vi "OpenByRefnumAndRunFP.vi"(0 "VI refnum":refnum<vi>, 5 "Wait until VI done?":bool caption="Wait until VI done? (F)", 7 "Auto dispose VI refnum?":bool=TRUE caption="Auto dispose VI refnum? (T)", 9 "Reentrancy mode":T2=enum."Auto" caption="Reentrancy mode (Auto)", 11 "Error in":errorcluster caption="Error in (no error)", 12 "Control names":string[](array[string]) caption="Control names (none)", 13 "Control values":variant[](array[variant]) caption="Control values (none)") -> (3 "VI refnum opened?":bool, 4 "VI refnum out":refnum<vi>, 6 "VI running?":bool, 8 "Last execution state":T1(ring), 10 "VI refnum opened as reentrant?":bool, 14 "Control values set?":bool, 15 "Error out":errorcluster)   [LabVIEW 2017, in "VILauncher.lvlib"]
doc: "Opens a reference to a dynamic VI either specified by path (<B>VI path</B>) or by reference (<B>VI refnum</B>), runs the dynamic VI, and returns the reference to it in <B>VI refnum out</B>.\n\nThis function will wait until the dynamic VI is done if <B>Wait until VI done?</B> is True (default is False), and it will auto dispose the dynamic VI reference (hand it over to the running dynamic VI) if <B>Auto dispose VI refnum?</B> is True. Note that if this function fails to run the dynamic VI, it will close the opened VI reference itself, in which case <B>VI refnum opened?</B> will be False and <B>VI refnum out</B> will be invalid.\n\nUse the optional <B>Reentrancy mode</B> input to specify whether the dynamic VI should be opened as a reentrant or a non-reentrant instance. Set this to Auto (default) to first try as reentrant, and if that fails, as non-reentrant. The <B>VI refnum opened as reentrant?</B> output will reflect the eventual instantiation mode.\n\nThe <B>VI running?</B> output will only be True if the dynamic VI's <B>Last execution state</B> is \"Run top level\". <B>VI running?</B> can be False even if the dynamic VI ran successfully - it might just have finished before this VI finished.\n\nOptionally you can send input data to the dynamic VI when running it using one of two modes; Right click this VI and use the Select Type menu to choose input data transfer mode:\n\nInput data via front panel\n-------------------------------\nSet data on the front panel of the dynamic VI before running it by wiring <B>Control names</B> and <B>Control values</B>. <B>Control values set?</B> will be True only if all <B>Control names</B> were valid.\n\nInput data via block diagram\n----------------------------------\nTransmit data to the dynamic VI after it has started by wiring <B>Input data names</B> and <B>Input data values</B>. If you use this mode the dynamic VI must use the WaitForInputData function to read the input data on the block diagram. The read in the dynamic VI must be finished before <B>Input data timeout</B> runs out. Set this timeout value to -1 (default) to wait indefinitely. If timeout does occur, <B>Input data timed out?</B> will be True. <B>Input data delivered?</B> will be True only if input data was in fact transmitted to the dynamic VI without any errors.\n\n<B>NOTE 1:</B> When using the 'Input data via block diagram' mode the dynamic VI must use the WaitForInputData function even if you send zero input data. To avoid this requirement for the dynamic VI when not passing any input data, please use the 'Input data via front panel' mode in this case.\n\n<B>NOTE 2:</B> The dynamic VI must have its front panel available at runtime for this function to work. The simplest way to ensure this, which also works in a built application without additional steps to be taken, is by enabling \"Show front panel when called\" in the \"Window Appearance\" section of the dynamic VI Properties.\n\nThis VI is reentrant, and it will only run if there is no error on <B>Error in</B>.\n\nSteen Schmidt\nGPower\n2/1 2013"
uses:
  VILauncher.lvlib
  Typedefs/ReentrancyMode.ctl
panel:
  # "Copyright © 2013\nGPower\nSee enclosed license file for terms and conditions"
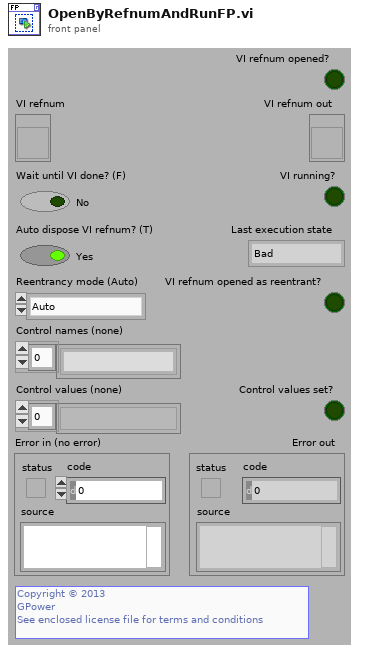
[diagram p1: front panel]
types:
  T1 = enum32{"Bad", "Idle", "Run top level", "Running"}
  T2 = typedef "VILauncher.lvlib/ReentrancyMode.ctl" = enum16{"Reentrant", "Non-reentrant", "Auto"}
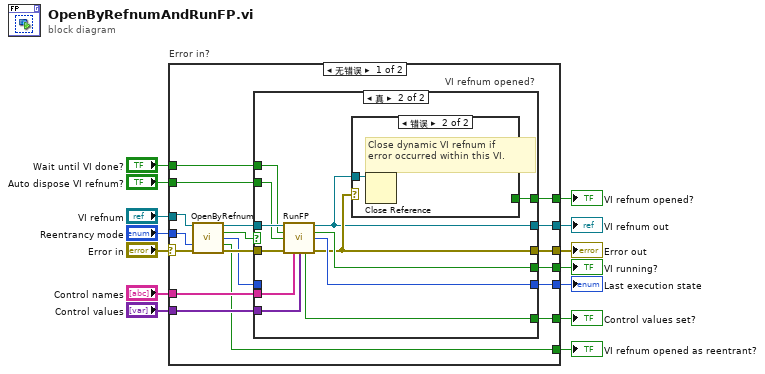
[diagram p0: block diagram]
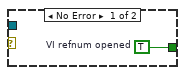
[diagram p3: hidden frame]
diagram:
  n1 = case "Error in?" shown="无错误" "Error in" {
    selector: "Error in" -> [w30 w50]
    tunnel: [w25 w50] -> w13
    tunnel: "Control names" -> [w32 _]
    tunnel: "Control values" -> [w31 _]
    tunnel: [w24 _] -> w10
    tunnel: "VI refnum" -> [w15 _]
    tunnel: "Reentrancy mode" -> [w28 _]
    tunnel: [w22 _] -> w8
    tunnel: "Auto dispose VI refnum?" -> [w21 _]
    tunnel: [w20 _] -> w6
    tunnel: [w19 _] -> w5
    tunnel: "Wait until VI done?" -> [w18 _]
    tunnel: [w17 _] -> w3
    tunnel: [w16 _] -> w2
    frame No Error {
      n2 = call "OpenByRefnum.vi"("VI refnum"=w15, "Reentrancy mode"=w28, "Error in"=w30) -> ("VI refnum out"=w26:refnum<vi>, "VI refnum opened?"=w27:bool, "Last execution state"=w23:T1, "VI refnum opened as reentrant?"=w22:bool, "Error out"=w29:errorcluster)  [unwired: 8 in]
      n3 = case "VI refnum opened?" shown="真" w27 {
        tunnel: w32 -> [_ w43]
        tunnel: w31 -> [_ w42]
        tunnel: w29 -> [w34 w47]
        tunnel: w26 -> [w35 w46]
        tunnel: [w34 w38] -> w25
        tunnel: [w35 w37] -> w24
        tunnel: w23 -> [w33 _]
        tunnel: w21 -> [_ w44]
        tunnel: [_ w39] -> w20
        tunnel: [w33 w40] -> w19
        tunnel: w18 -> [_ w45]
        tunnel: [_ w41] -> w17
        tunnel: [_ w36] -> w16
        frame False {
        }
        frame True {
          n4 = call "RunFP.vi"("VI refnum in"=w46, "Wait until VI done?"=w45, "Auto dispose VI refnum?"=w44, "Error in"=w47, "Control names"=w43, "Control values"=w42) -> ("VI refnum out"=w37:refnum<vi>, "VI running?"=w39:bool, "Last execution state"=w40:T1, "Control values set?"=w41:bool, "Error out"=w38:errorcluster)  [unwired: 5 in]
          n5 = case shown="错误" w38 {
            tunnel: w37 -> [_ w49]
            tunnel: [w48 _] -> w36
            frame No Error {
              w48 = TRUE  # VI refnum opened
            }
            frame Error {
              # "Close dynamic VI refnum if\nerror occurred within this VI."
              n6 = Close Reference(reference=w49) -> ()  [unwired: 1 in, 1 out]
            }
          }
        }
      }
    }
    frame Error {
    }
  }
  "Error out" <- w13
  "VI refnum out" <- w10
  "VI running?" <- w6
  "VI refnum opened as reentrant?" <- w8
  "Last execution state" <- w5
  "Control values set?" <- w3
  "VI refnum opened?" <- w2
